vi "Manual Triggered B-Scan 2.vi"() -> ()   [LabVIEW 2012]
uses:
  LabVIEW/user.lib/SpectralRadar.llb/Processing Flag Selection.ctl
  LabVIEW/user.lib/SpectralRadar.llb/set Scan Output.vi
  LabVIEW/user.lib/SpectralRadar.llb/display Data 2D.vi
  LabVIEW/user.lib/SpectralRadar.llb/OCT Device.lvclass
  LabVIEW/user.lib/SpectralRadar.llb/Processing.lvclass
  LabVIEW/user.lib/SpectralRadar.llb/Raw Data.lvclass
  LabVIEW/user.lib/SpectralRadar.llb/Data.lvclass
panel:
  in  "stop":bool
  out "B-scan display":dbl[][](graph)
  in  "A-scans / B-scan":i32=512
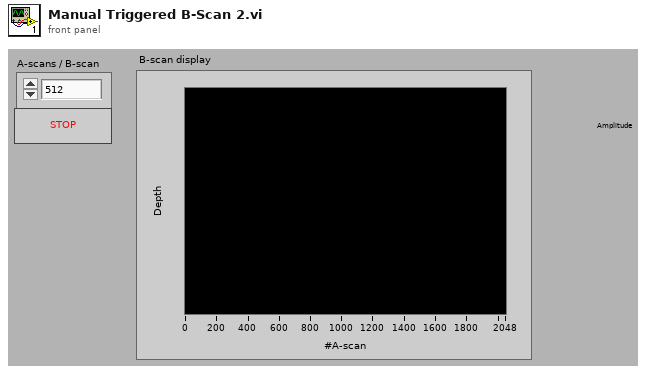
[diagram p1: front panel]
types:
  T1 = typedef "Processing.lvclass/Processing Flag Selection.ctl" = enum16{"Use Offset Errors", "Remove DC Spectrum", "Remove Advanced DC Spectrum", "Use Apodization", "Use Scan For Apodization", "Filter Undersampled Signals", "Use Dispersion Compensation", "Use Dechirp", "Use Extended Adjust", "Full Range Output", "Filter DC", "Autocorrelation Compensation", "DEFR", "Only Windowing", "Remove Fixed Pattern"}
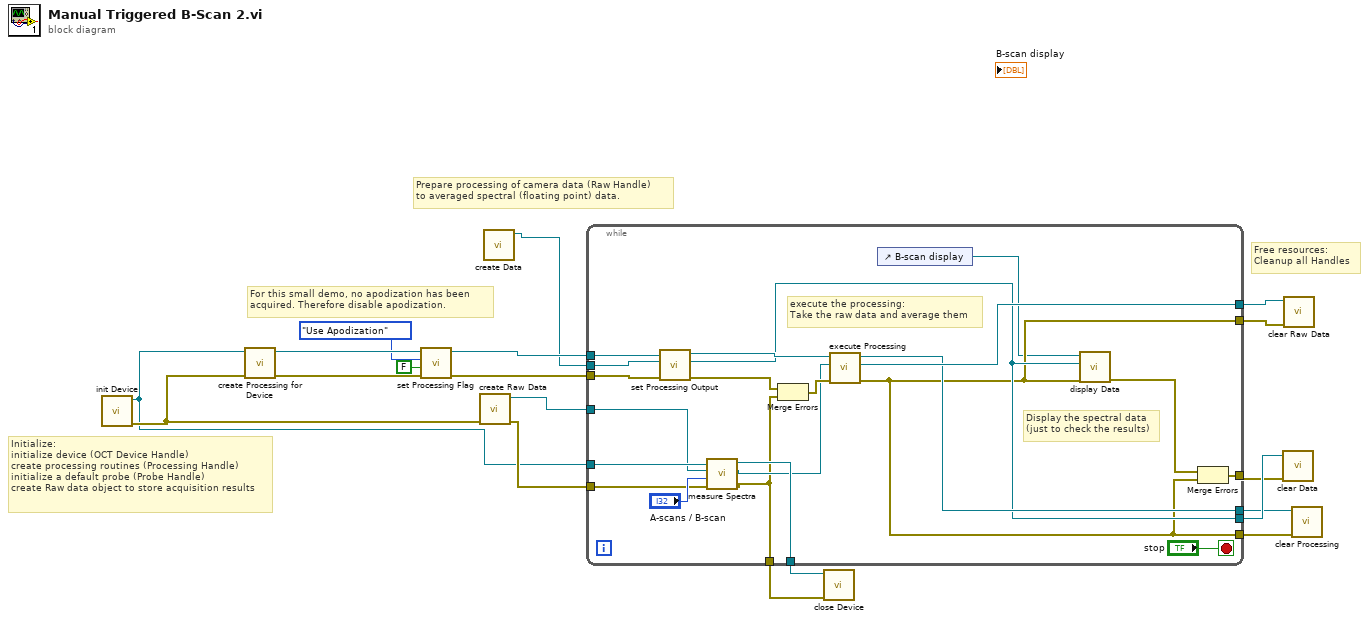
[diagram p0: block diagram]
diagram:
  # "For this small demo, no apodization has been \nacquired. Therefore disable apodization."
  # "Free resources:\nCleanup all Handles"
  # "Prepare processing of camera data (Raw Handle)\nto averaged spectral (floating point) data."
  # "Initialize:\ninitialize device (OCT Device Handle)\ncreate processing routines (Processing Handle)\ninitialize a default probe (Probe Handle)\ncreate Raw data object to store acquisition results"
  n1 = call "init Device.vi"() -> ("error out"=w19:errorcluster, "OCTDevice"=w6:refnum<class "OCT Device.lvclass">)  [unwired: 6 in]
  n2 = call "create Processing for Device.vi"("error in (no error)"=w19, "OCTDevice"=w6) -> ("error out"=w9:errorcluster, "Processing"=w15:refnum<class "Processing.lvclass">)  [unwired: 3 in, 1 out]
  n3 = call "set Processing Flag.vi"("error in (no error)"=w9, "Flag"=FALSE, "Processing Flag Selection"=Processing_Flag_Selection."Use Apodization", "Processing"=w15) -> ("error out"=w12:errorcluster, "Processing"=w14:refnum<class "Processing.lvclass">)  [unwired: 2 in]
  n4 = call "create Raw Data.vi"("error in (no error)"=w19) -> ("error out"=w7:errorcluster, "Raw Data"=w18:refnum<class "Raw Data.lvclass">)  [unwired: 5 in]
  n5 = call "create Data.vi"() -> ("Data"=w3:refnum<class "Data.lvclass">)  [unwired: 6 in, 1 out]
  n6 = while {
    tunnel: w18 -> [w27]
    tunnel: w3 -> [w40]
    tunnel: w6 -> [w28]
    tunnel: [w38] -> w17
    tunnel: [w36] -> w4
    tunnel: [w26] -> w11
    tunnel: [w24] -> w10
    tunnel: [w33] -> w2
    tunnel: [w32] -> w5
    tunnel: [w29] -> w16
    tunnel: w14 -> [w31]
    tunnel: w12 -> [w30]
    tunnel: [w29] -> w1
    tunnel: w7 -> [w22]
    stop <- "stop" stop-if-true
    # "Display the spectral data\n(just to check the results)"
    # "execute the processing:\nTake the raw data and average them"
    n7 = call-poly "set Processing Output.vi"("error in (no error)"=w30, "Data"=w40, "Processing"=w31) -> ("error out"=w35:errorcluster, "Data"=w32:refnum<class "Data.lvclass">, "Processing"=w39:refnum<class "Processing.lvclass">)  [unwired: 2 in]
    n8 = call "measure Spectra.vi"("error in (no error)"=w22, "NumberOfSpectra"="A-scans / B-scan", "Raw Data"=w27, "OCTDevice"=w28) -> ("error out"=w24:errorcluster, "Raw Data"=w25:refnum<class "Raw Data.lvclass">, "OCTDevice"=w26:refnum<class "OCT Device.lvclass">)  [unwired: 2 in]
    n9 = Merge Errors(w35, w24) -> (w34:errorcluster)
    n10 = call "execute Processing.vi"("error in (no error)"=w34, "Raw Data"=w25, "Processing"=w39) -> ("error out"=w29:errorcluster, "Raw Data"=w38:refnum<class "Raw Data.lvclass">, "Processing"=w33:refnum<class "Processing.lvclass">)  [unwired: 2 in]
    n11 = control-ref of="B-scan display"() -> (w21:refnum<vi>)
    n12 = call-poly "display Data.vi"("error in (no error)"=w29, "Data in"=w32, "IntGraph Refnum"=w21) -> ("error out"=w37:errorcluster)  [unwired: 2 in, 2 out]
    n13 = Merge Errors(w37, w29) -> (w36:errorcluster)
  }
  n14 = call "close Device.vi"("error in (no error)"=w10, "OCTDevice"=w11) -> ()  [unwired: 5 in, 1 out]
  n15 = call "clear Data.vi"("error in (no error)"=w4, "Data"=w5) -> ()  [unwired: 5 in, 1 out]
  n16 = call "clear Raw Data.vi"("error in (no error)"=w16, "Raw Data"=w17) -> ()  [unwired: 5 in, 1 out]
  n17 = call "clear Processing.vi"("error in (no error)"=w1, "Processing"=w2) -> ()  [unwired: 5 in, 1 out]
